vi "Intake_Disc_Execute.vi"() -> ()   [LabVIEW 2018]
uses:
  <vilib>/Rock Robotics/WPI/Solenoid/WPI_SolenoidValue.ctl
  <vilib>/Rock Robotics/WPI/DriverStation/WPI_DriverStationRobotMode2.ctl
  Global_Variables/Intake_Disc_Globals.vi
  Global_Variables/Robot_Global_Data.vi
  Global_Variables/Elevator_Globals.vi
  Global_Variables/Autonomous_Globals.vi
  <vilib>/Rock Robotics/WPI/Solenoid/WPI_SolenoidSetEnum.vi
  Global_Variables/LED_Globals.vi
panel:
  out "Numeric":i32
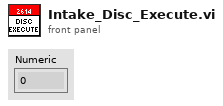
[diagram p1: front panel]
types:
  T1 = typedef "WPI_SolenoidValue.ctl" = enum16{"Off", "On", "Forward", "Reverse"}
  T2 = typedef "WPI_SolenoidDevRef.ctl" = cluster{"DevStatus":errorcluster, "Pneumatics Control Module":u8, "Forward Solenoid Channel":T3, "Reverse Solenoid Channel":T3}
  T3 = typedef "WPI_SolenoidChannel.ctl" = enum8{"Solenoid 0", "Solenoid 1", "Solenoid 2", "Solenoid 3", "Solenoid 4", "Solenoid 5", "Solenoid 6", "Solenoid 7", "Invalid"}
  T4 = typedef "WPI_DriverStationRobotMode2.ctl" = enum16{"Autonomous Disabled", "Autonomous Enabled", "Teleop Disabled", "Teleop Enabled", "Disconnected", "Finish", "Test Disabled", "Test Enabled", "Emergency Stopped"}
  T5 = typedef "Intake_Disc_Notifier.ctl" = cluster{"Intake_Disc_Control_Type":T6, "Manual_Disc_Toggle":bool, "Disc_Toggle":bool, "Disc_Toggle_State":bool, "Manual_Press_Toggle":bool, "Disc_Press_State":bool, "Press_Toggle":bool, "Press_Pnuematic":T1, "Disc_Pnuematic":T1, "Disc_Notifier":refnum<notifier>, "Step":i32}
  T6 = typedef "Intake_Disc_Control_Type.ctl" = enum16{"No_Op", "Manual_Disc_Toggle", "Disc_Toggle", "Manual_Press_Toggle", "Press_Toggle", "Acquire_Hatch", "Retract"}
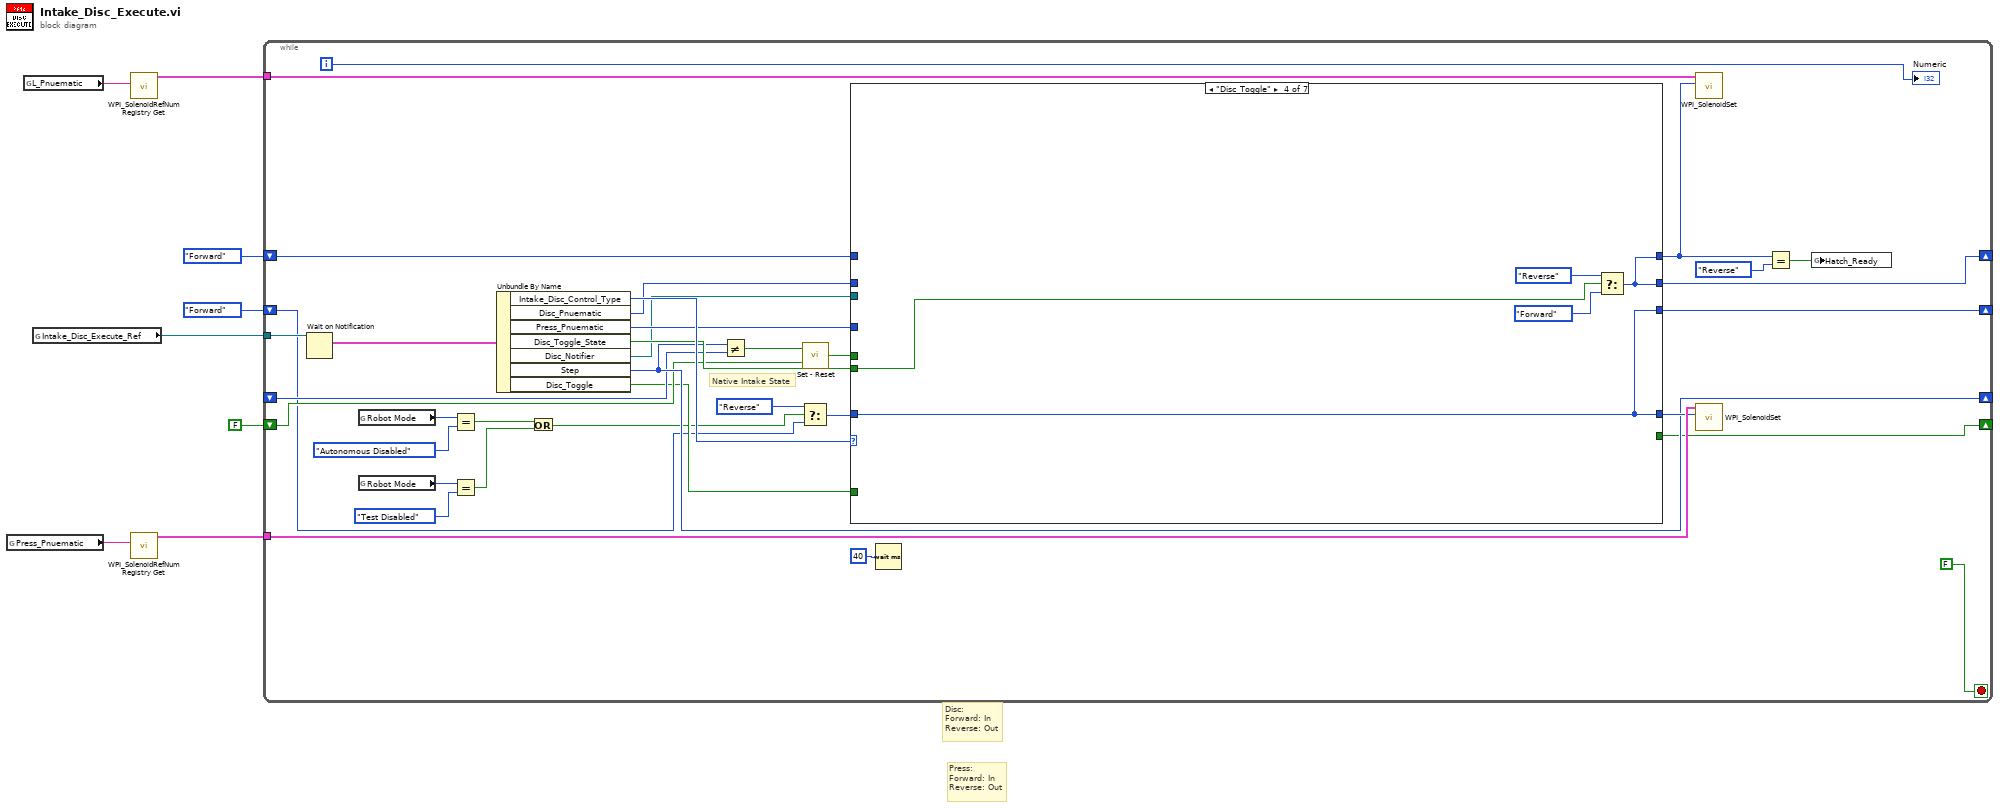
[diagram p0: block diagram]
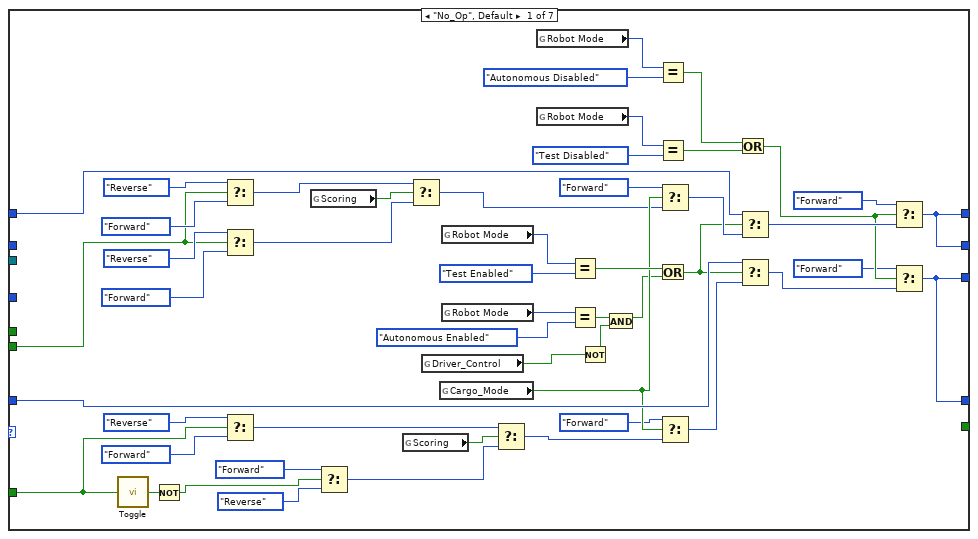
[diagram p2: hidden frame]
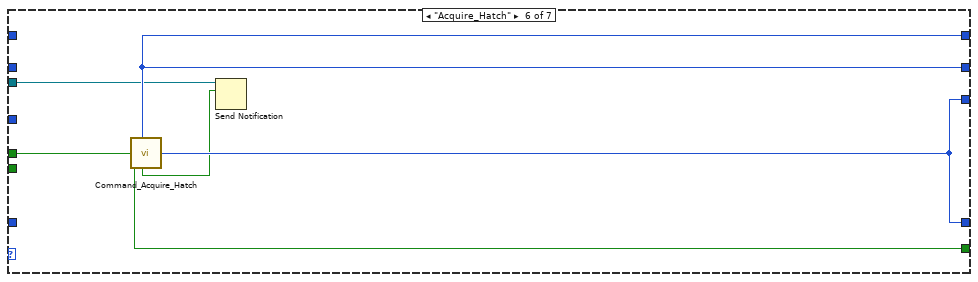
[diagram p6: hidden frame]
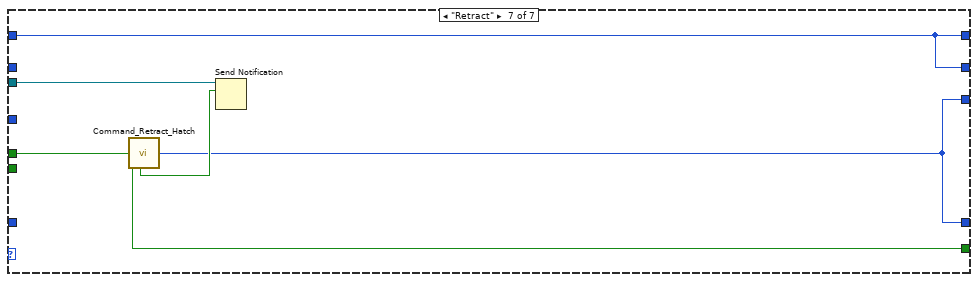
[diagram p7: hidden frame]
diagram:
  # "Press:\nForward: In \nReverse: Out"
  # "Disc:\nForward: In \nReverse: Out"
  n1 = global read "Intake_Disc_Globals.vi" "Press_Pnuematic"() -> (w3:string)
  n2 = global read "Intake_Disc_Globals.vi" "L_Pnuematic"() -> (w7:string)
  n3 = global read "Intake_Disc_Globals.vi" "Intake_Disc_Execute_Ref"() -> (w8:refnum<notifier>)
  n4 = call <vilib>:"WPI_SolenoidRefNum Registry Get.vi"("refnum name"=w7) -> ("SolenoidDevRef"=w6:T2)  [unwired: 9 in, 1 out]
  n5 = call <vilib>:"WPI_SolenoidRefNum Registry Get.vi"("refnum name"=w3) -> ("SolenoidDevRef"=w2:T2)  [unwired: 9 in, 1 out]
  n6 = while {
    tunnel: w8 -> [w41]
    tunnel: w6 -> [w40]
    shift-right: [w38] -> _
    shift-left: WPI_SolenoidValue."Forward" ("Value") -> [w39]
    shift-right: [w31] -> _
    shift-left: WPI_SolenoidValue."Forward" ("Value") -> [w14]
    tunnel: w2 -> [w33]
    shift-right: [w27] -> _
    shift-left: _ -> [w26]
    shift-right: [w25] -> _
    shift-left: FALSE ("Reint") -> [w22]
    i -> [w20]
    stop <- FALSE stop-if-true
    # "Native Intake State"
    n7 = Wait on Notification(notifier=w41) -> (notification=w43:T5)  [unwired: 3 in, 3 out]
    n8 = global read "Robot_Global_Data.vi" "Robot Mode"() -> (w11:T4)
    n9 = global read "Robot_Global_Data.vi" "Robot Mode"() -> (w16:T4)
    n10 = Equal?(x=w11, y=WPI_DriverStationRobotMode2."Autonomous Disabled") -> (x = y?=w9:bool)
    n11 = Equal?(x=w16, y=WPI_DriverStationRobotMode2."Test Disabled") -> (x = y?=w13:bool)
    n12 = Unbundle By Name(w43) -> ("Intake_Disc_Control_Type"=w42:T6, "Disc_Pnuematic"=w30:T1, "Press_Pnuematic"=w34:T1, "Disc_Toggle_State"=w29:bool, "Disc_Notifier"=w28:refnum<notifier>, "Step"=w27:i32, "Disc_Toggle"=w21:bool)
    n13 = Or(x=w9, y=w13) -> (x .or. y?=w12:bool)
    n14 = Not Equal?(x=w27, y=w26) -> (x != y?=w24:bool)
    n15 = Select(t=WPI_SolenoidValue."Reverse", s=w12, f=w14) -> (s? t:f=w17:T1)
    n16 = call "Set - Reset.vi"("Reset"=w22, "Set"=w24) -> ("Output"=w23:bool)
    n17 = case shown="\"Disc_Toggle\"" w42 {
      tunnel: [w61 w95 w98 w102 w105 w111 w112] -> w37
      tunnel: w39 -> [w92 _ w98 _ w105 _ w112]
      tunnel: [w61 w95 w98 w102 w105 w111 w112] -> w38
      tunnel: w30 -> [_ w95 _ _ _ _ _]
      tunnel: w34 -> [_ _ w97 _ w104 _ _]
      tunnel: [w59 w96 w97 w103 w104 w110 w113] -> w32
      tunnel: [w59 w96 w97 w103 w104 w110 w113] -> w31
      tunnel: w17 -> [w90 w96 _ w103 _ _ _]
      tunnel: w29 -> [w68 _ _ w99 _ _ _]
      tunnel: w28 -> [_ _ _ _ _ w108 w117]
      tunnel: w23 -> [_ _ _ _ _ w107 w114]
      tunnel: [_ _ _ _ _ w106 w115] -> w25
      tunnel: w21 -> [w66 _ _ _ _ _ _]
      frame "No_Op", Default {
        n18 = call "Toggle.vi"("Boolean"=w66) -> ("Boolean Out"=w67:bool)
        n19 = Not(x=w67) -> (.not. x?=w49:bool)
        n20 = Select(t=WPI_SolenoidValue."Reverse" ("y"), s=w68, f=WPI_SolenoidValue."Forward" ("y")) -> (s? t:f=w80:T1)
        n21 = Select(t=WPI_SolenoidValue."Reverse" ("y"), s=w68, f=WPI_SolenoidValue."Forward" ("y")) -> (s? t:f=w79:T1)
        n22 = Select(t=WPI_SolenoidValue."Reverse", s=w66, f=WPI_SolenoidValue."Forward" ("y")) -> (s? t:f=w78:T1)
        n23 = global read "Elevator_Globals.vi" "Scoring"() -> (w82:bool)
        n24 = Select(t=WPI_SolenoidValue."Forward" ("y"), s=w49, f=WPI_SolenoidValue."Reverse" ("y")) -> (s? t:f=w77:T1)
        n25 = global read "Elevator_Globals.vi" "Scoring"() -> (w81:bool)
        n26 = Select(t=w80, s=w82, f=w79) -> (s? t:f=w84:T1)
        n27 = global read "Autonomous_Globals.vi" "Driver_Control"() -> (w45:bool)
        n28 = global read "Intake_Disc_Globals.vi" "Cargo_Mode"() -> (w87:bool)
        n29 = global read "Robot_Global_Data.vi" "Robot Mode"() -> (w94:T4)
        n30 = global read "Robot_Global_Data.vi" "Robot Mode"() -> (w63:T4)
        n31 = Select(t=w78, s=w81, f=w77) -> (s? t:f=w83:T1)
        n32 = global read "Robot_Global_Data.vi" "Robot Mode"() -> (w56:T4)
        n33 = global read "Robot_Global_Data.vi" "Robot Mode"() -> (w54:T4)
        n34 = Equal?(x=w94, y=WPI_DriverStationRobotMode2."Test Enabled") -> (x = y?=w91:bool)
        n35 = Equal?(x=w63, y=WPI_DriverStationRobotMode2."Autonomous Enabled") -> (x = y?=w47:bool)
        n36 = Not(x=w45) -> (.not. x?=w46:bool)
        n37 = And(x=w47, y=w46) -> (x .and. y?=w48:bool)
        n38 = Equal?(x=w56, y=WPI_DriverStationRobotMode2."Autonomous Disabled") -> (x = y?=w58:bool)
        n39 = Equal?(x=w54, y=WPI_DriverStationRobotMode2."Test Disabled") -> (x = y?=w55:bool)
        n40 = Or(x=w91, y=w48) -> (x .or. y?=w65:bool)
        n41 = Select(t=WPI_SolenoidValue."Forward" ("y"), s=w87, f=w84) -> (s? t:f=w89:T1)
        n42 = Select(t=WPI_SolenoidValue."Forward" ("y"), s=w87, f=w83) -> (s? t:f=w88:T1)
        n43 = Or(x=w58, y=w55) -> (x .or. y?=w52:bool)
        n44 = Select(t=w92, s=w65, f=w89) -> (s? t:f=w62:T1)
        n45 = Select(t=w90, s=w65, f=w88) -> (s? t:f=w60:T1)
        n46 = Select(t=WPI_SolenoidValue."Forward", s=w52, f=w62) -> (s? t:f=w61:T1)
        n47 = Select(t=WPI_SolenoidValue."Forward", s=w52, f=w60) -> (s? t:f=w59:T1)
      }
      frame "Manual_Disc_Toggle" {
      }
      frame "Manual_Press_Toggle" {
      }
      frame "Disc_Toggle" {
        n48 = Select(t=WPI_SolenoidValue."Reverse" ("Value"), s=w99, f=WPI_SolenoidValue."Forward" ("Value")) -> (s? t:f=w102:T1)
      }
      frame "Press_Toggle" {
      }
      frame "Acquire_Hatch" {
        n49 = call "Command_Acquire_Hatch.vi"("Startup"=w107) -> ("Disc"=w111:T1, "Reint"=w106:bool, "Completed"=w109:bool, "Press"=w110:T1)  [unwired: 1 in]
        n50 = Send Notification(notification=w109, notifier=w108) -> ()  [unwired: 1 in, 2 out]
      }
      frame "Retract" {
        n51 = call "Command_Retract_Hatch.vi"("Startup"=w114) -> ("Reint"=w115:bool, "Completed"=w116:bool, "Press"=w113:T1)  [unwired: 2 in]
        n52 = Send Notification(notification=w116, notifier=w117) -> ()  [unwired: 1 in, 2 out]
      }
    }
    n53 = Wait (ms)(milliseconds to wait=u32 40) -> ()  [unwired: 1 out]
    n54 = call-poly <vilib>:"WPI_SolenoidSet.vi"("Value"=w37, "SolenoidDevRef"=w40) -> ()  [unwired: 8 in, 2 out]
    n55 = call-poly <vilib>:"WPI_SolenoidSet.vi"("Value"=w32, "SolenoidDevRef"=w33) -> ()  [unwired: 8 in, 2 out]
    n56 = Equal?(x=w37, y=WPI_SolenoidValue."Reverse") -> (x = y?=w36:bool)
    n57 = global write "LED_Globals.vi" "Hatch_Ready"(w36) -> ()
    "Numeric" <- w20
  }
